vi "Show Configuration List Error Dialog.vi"(8 "error in (no error)":errorcluster, 10 "Value":path, 11 "UI in":refnum<class "UI.lvclass">) -> (0 "error out":errorcluster)   [LabVIEW 2020, in "AR Example.lvlib" / "UI.lvclass"]
uses:
  UI.lvclass
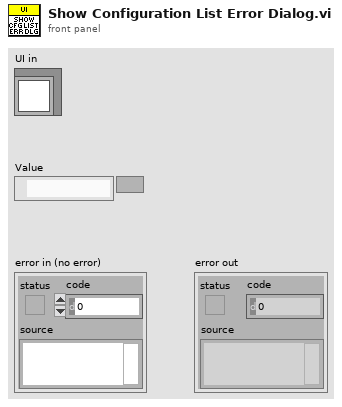
[diagram p1: front panel]
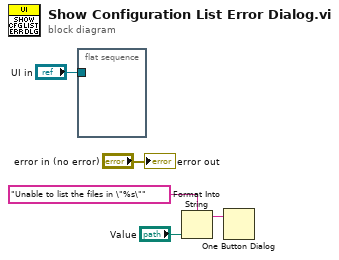
[diagram p0: block diagram]
diagram:
  n1 = flat-sequence {
    tunnel: "UI in" -> [_]
    frame #0 {
    }
  }
  n2 = Format Into String(format string="Unable to list the files in \"%s\"", "Value") -> (resulting string=w2:string)  [unwired: 2 in, 1 out]
  n3 = One Button Dialog(message=w2) -> ()  [unwired: 1 in, 1 out]
  "error out" <- "error in (no error)"
